vi "SetParameter.vi"(8 "error in (no error)":errorcluster, 9 "Value":string, 10 "ID":u16, 11 "ZWO_ASI in":refnum<class "ZWO_ASI.lvclass">) -> (0 "error out":errorcluster, 3 "ZWO_ASI out":refnum<class "ZWO_ASI.lvclass">)   [LabVIEW 2023, in "ZWO_ASI.lvlib" / "ZWO_ASI.lvclass"]
uses:
  ZWO_ASI.lvclass
  ZWO_ASI.lvclass/ZWO_ASI.ctl
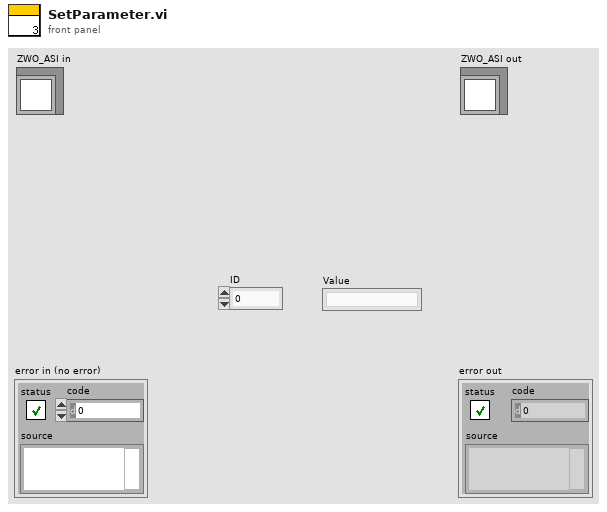
[diagram p1: front panel]
types:
  T1 = cluster{"name":string, "ControlType":u32, "plValue out":i32, "MaxValue":i32, "MinValue":i32}[]
  T2 = cluster{"name":string, "ControlType":u32, "plValue out":i32, "MaxValue":i32, "MinValue":i32}
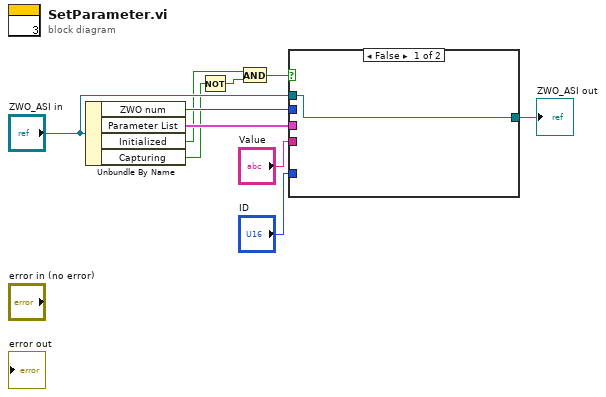
[diagram p0: block diagram]
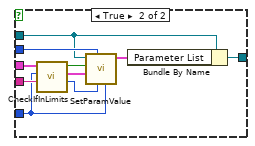
[diagram p2: hidden frame]
diagram:
  n1 = Unbundle By Name("ZWO_ASI in") -> ("ZWO num"=w9:i32, "Parameter List"=w7:T1, "Initialized"=w4:bool, "Capturing"=w2:bool)
  n2 = Not(x=w2) -> (.not. x?=w3:bool)
  n3 = And(x=w4, y=w3) -> (x .and. y?=w1:bool)
  n4 = case shown="False" w1 {
    tunnel: "Value" -> [_ w21]
    tunnel: w9 -> [_ w17]
    tunnel: "ID" -> [_ w16]
    tunnel: w7 -> [_ w15]
    tunnel: "ZWO_ASI in" -> [w11 w13]
    tunnel: [w11 w12] -> w5
    frame False {
    }
    frame True {
      n5 = call "CheckIfInLimits.vi"("Value"=w21, "ID"=w16, "Parameter List"=w15) -> ("plValue"=w20:i32, "Cluster"=w19:T2, "Boolean"=w18:bool)  [unwired: 6 in]
      n6 = call "SetParamValue.vi"("ID"=w16, "plValue"=w20, "ZWO num"=w17, "Cluster"=w19, "Boolean"=w18, "ZWO_ASI in"=w13) -> ("Parameter List"=w14:T1)  [unwired: 5 in]
      n7 = Bundle By Name(cluster=w13, "Parameter List"=w14) -> (w12:refnum<class "ZWO_ASI.lvclass">)
    }
  }
  "ZWO_ASI out" <- w5
